vi "Serial.vi"(6 "Function Choose":enum16{"Init", "Write", "Read", "Close"}(ring), 8 "error in (no error)":errorcluster, 9 "baud rate (9600)":u32=115200, 10 "write buffer":string, 11 "VISA resource name":refnum<visa-resource-name>) -> (0 "error out":errorcluster, 2 "Result":string, 3 "VISA resource name 2":refnum<visa-resource-name>)   [LabVIEW 2020]
uses:
  <vilib>/Instr/_visa.llb/VISA Configure Serial Port (Instr).vi
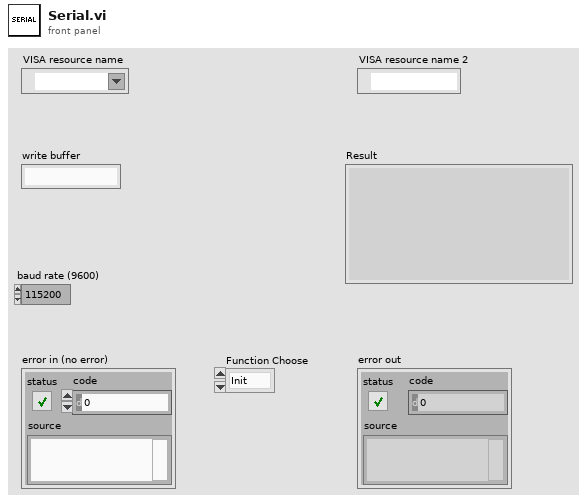
[diagram p1: front panel]
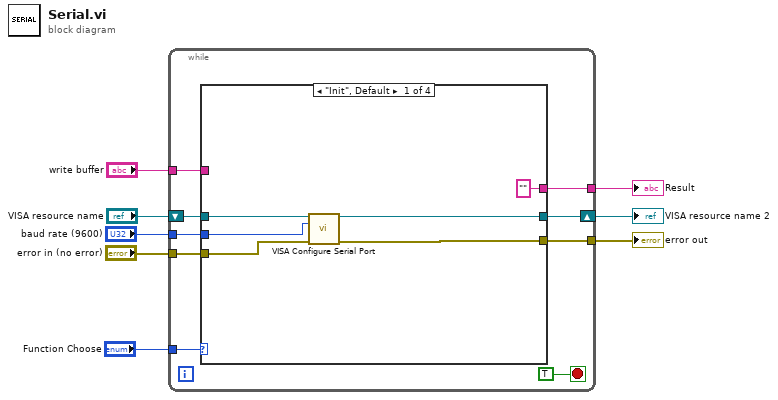
[diagram p0: block diagram]
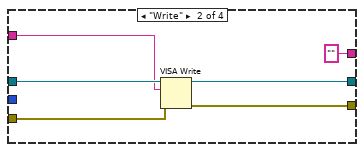
[diagram p2: hidden frame]
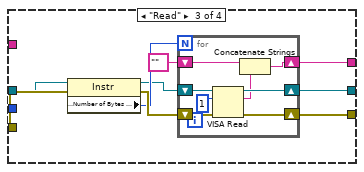
[diagram p3: hidden frame]
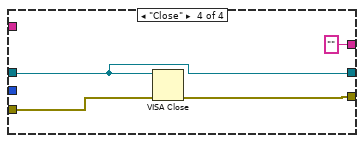
[diagram p4: hidden frame]
diagram:
  n1 = while {
    tunnel: "Function Choose" -> [w17]
    tunnel: "error in (no error)" -> [w16]
    shift-right: [w12] -> w2
    shift-left: "VISA resource name" -> [w14]
    tunnel: [w13] -> w5
    tunnel: [w11] -> w4
    tunnel: "write buffer" -> [w10]
    tunnel: "baud rate (9600)" -> [w9]
    stop <- TRUE stop-if-true
    n2 = case shown="\"Init\", Default" w17 {
      tunnel: w16 -> [w23 w29 w38 w50]
      tunnel: [w21 w26 w34 w49] -> w11
      tunnel: [w20 w27 w33 w48] -> w12
      tunnel: w14 -> [w22 w28 w32 w48]
      tunnel: ["" "" w30 ""] -> w13
      tunnel: w10 -> [_ w24 _ _]
      tunnel: w9 -> [w18 _ _ _]
      frame "Init", Default {
        n3 = call-poly "VISA Configure Serial Port"("VISA resource name"=w22, "baud rate (9600)"=w18, "error in (no error)"=w23) -> ("VISA resource name out"=w20:refnum<visa-resource-name>, "error out"=w21:errorcluster)  [unwired: 11 in]
      }
      frame "Write" {
        n4 = VISA Write(VISA resource name=w28, write buffer=w24, error in (no error)=w29) -> (VISA resource name out=w27:refnum<visa-resource-name>, error out=w26:errorcluster)  [unwired: 1 out]
      }
      frame "Read" {
        n5 = property class="Instr"(reference=w32, error in=w38) -> (reference out=w35:refnum<visa-resource-name>, error out=w37:errorcluster, "Serial Settings:Number of Bytes at Serial Port"=w36:u32)
        n6 = for {
          N: w36 -> [_]
          shift-right: [w42] -> w33
          shift-left: w35 -> [w44]
          shift-right: [w39] -> w30
          shift-left: "" -> [w40]
          shift-right: [w43] -> w34
          shift-left: w37 -> [w45]
          n7 = VISA Read(VISA resource name=w44, byte count=u32 1, error in (no error)=w45) -> (VISA resource name out=w42:refnum<visa-resource-name>, read buffer=w41:string, error out=w43:errorcluster)  [unwired: 1 out]
          n8 = Concatenate Strings(w40, w41) -> (w39:string)
        }
      }
      frame "Close" {
        n9 = VISA Close(VISA resource name=w48, error in (no error)=w50) -> (error out=w49:errorcluster)
      }
    }
  }
  "Result" <- w5
  "error out" <- w4
  "VISA resource name 2" <- w2
